vi "AnalyseFeRfe.vi"(6 "NISTData.NIDataArray":T2 {"Time Stamp" format="%^<%.3X\n%x>T"}, 8 "error in (no error)":errorcluster, 10 "Fluke":dbl[][](array[numeric]), 11 "NIST":dbl[][](array[numeric])) -> (0 "error out":errorcluster, 2 "Plot":cluster{dbl, "Time":dbl, dbl[][]}[](array[cluster]), 3 "FERfe Stats":dbl[][](array[numeric]))   [LabVIEW 2014]
uses:
  typedefs/NIDataArray.ctl
  typedefs/NIData.ctl
  typedefs/PhasorRectangular.ctl
  <vilib>/Analysis/6fits.llb/Curve Fitting Criteria.ctl
  <vilib>/measure/matone.llb/Extract Single Tone Information 1 Chan.vi
  <vilib>/Analysis/NI_AALPro.lvlib
  <vilib>/measure/NI_MAPro.lvlib
  <vilib>/Analysis/NI_AALBase.lvlib
panel:
  out "RFE Residual":T1(graph)
  out "FE Residual":T1(graph)
  out "RFE":cluster{dbl, "Time":dbl, dbl[][]}(graph)
  out "FE":cluster{dbl, "Time":dbl, dbl[][]}(graph)
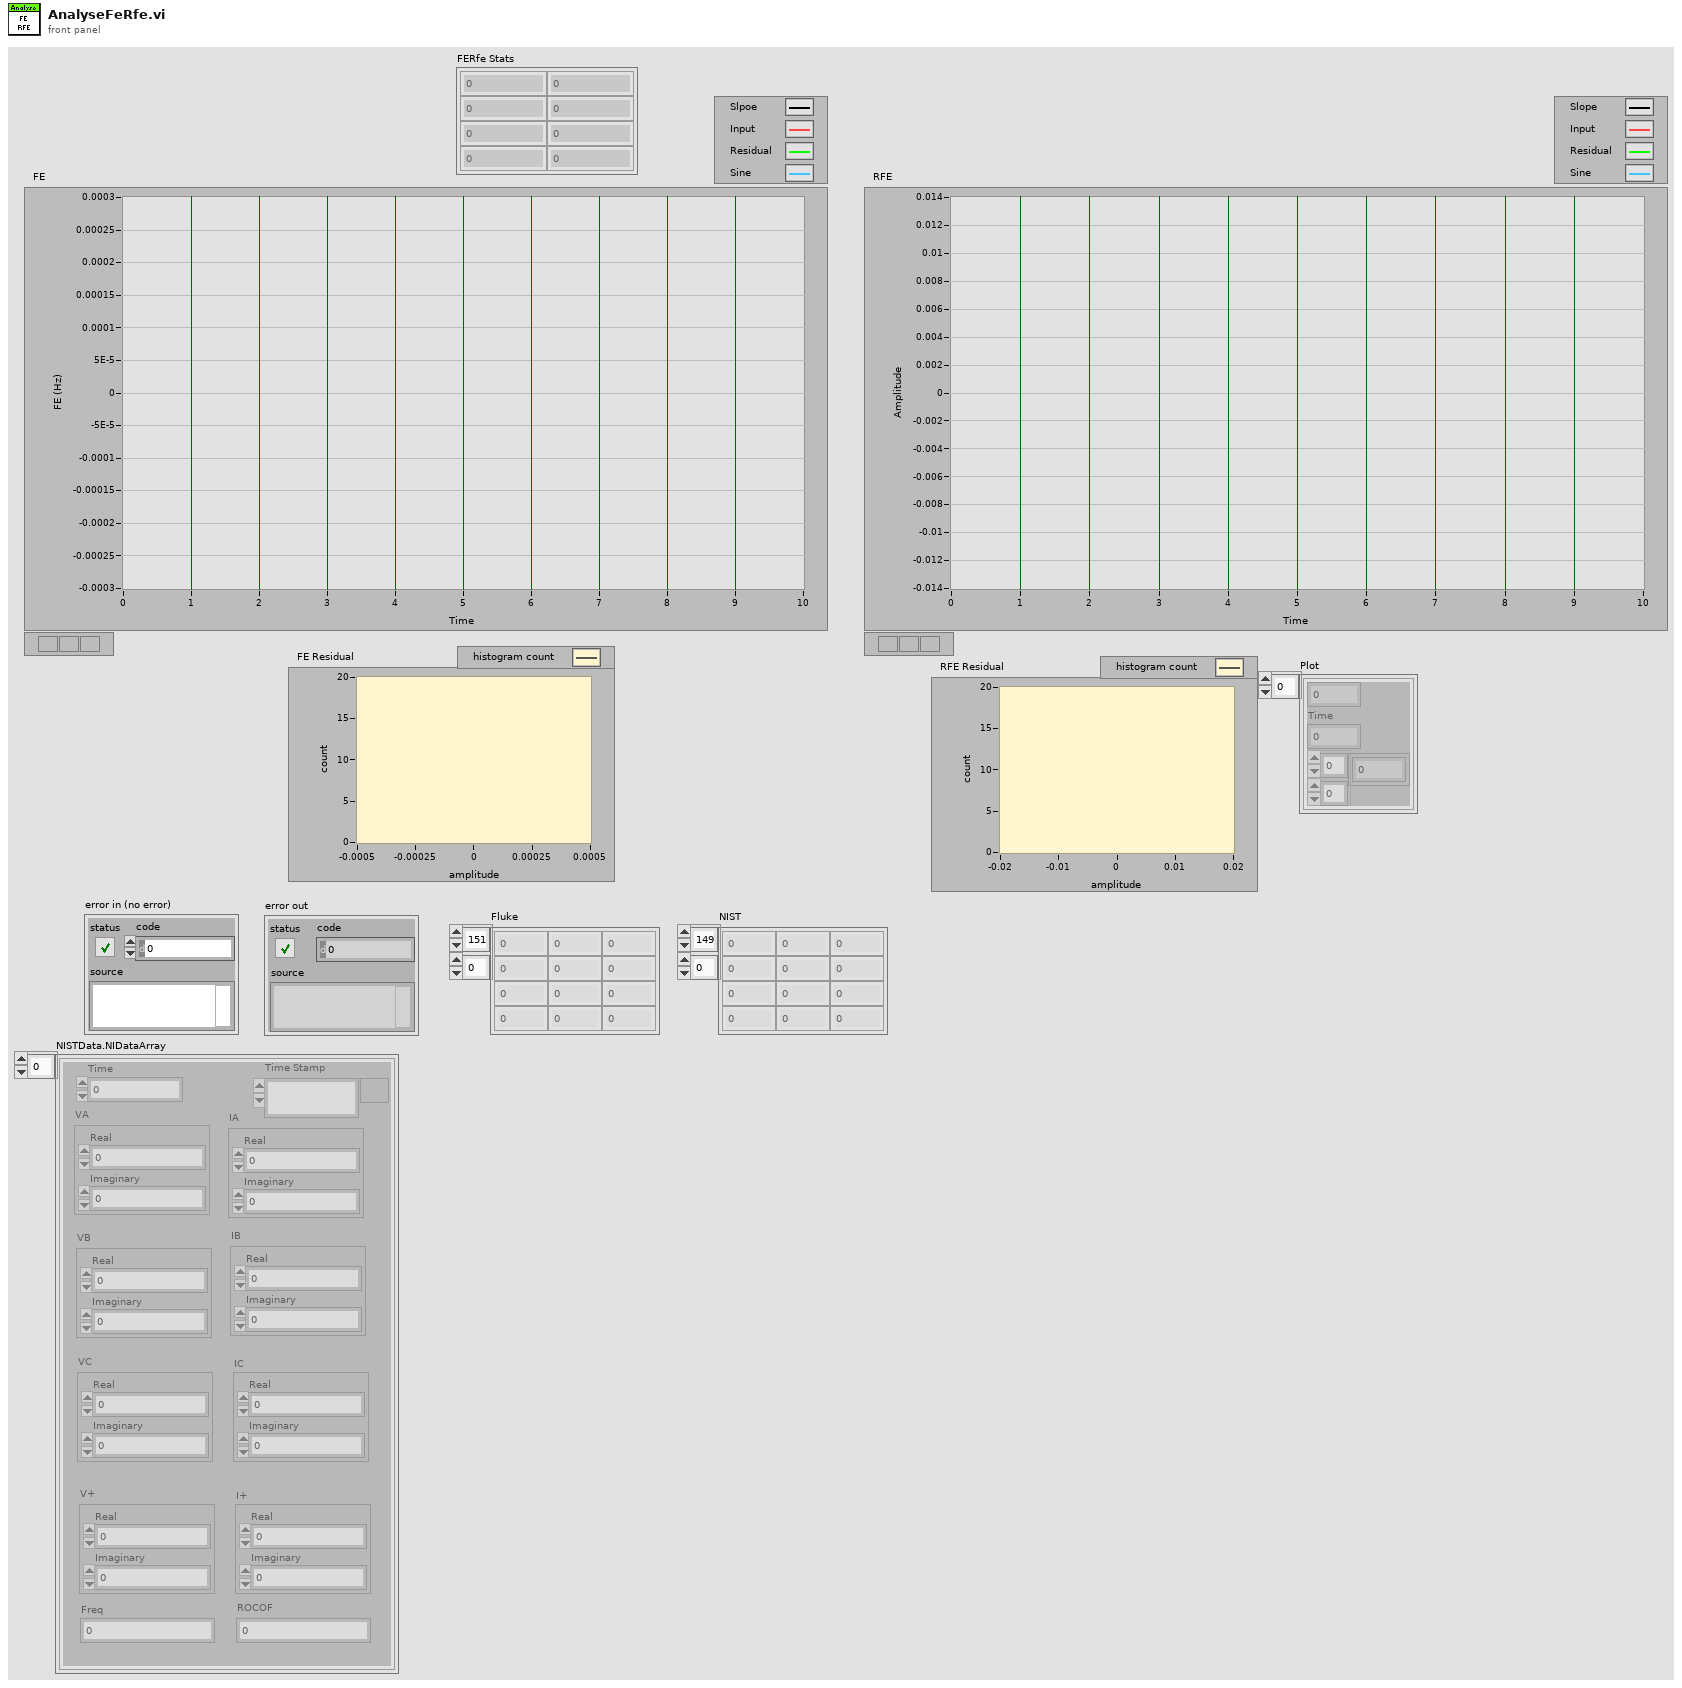
[diagram p1: front panel]
types:
  T1 = cluster{"X Values":dbl[], "Histogram: h(x)":i32[]}
  T2 = typedef "NIDataArray.ctl" = T3[]
  T3 = typedef "NIData.ctl" = cluster{"Time":dbl, "VA":T4, "VB":T4, "VC":T4, "V+":T4, "IA":T4, "IB":T4, "IC":T4, "I+":T4, "Freq":dbl, "ROCOF":dbl, "Time Stamp":timestamp}
  T4 = typedef "PhasorRectangular.ctl" = cluster{"Real":dbl, "Imaginary":dbl}
  T5 = enum32{"none", "input signal", "detected signal", "residual signal"}
  T6 = typedef "NI_AALPro.lvlib/Curve Fitting Criteria.ctl" = u16
  T7 = cluster{"exported time signal":waveform(dbl), "exported spectrum (dB)":cluster{"f0":dbl, "df":dbl, "dB Spectrum (Hann)":dbl[]}}
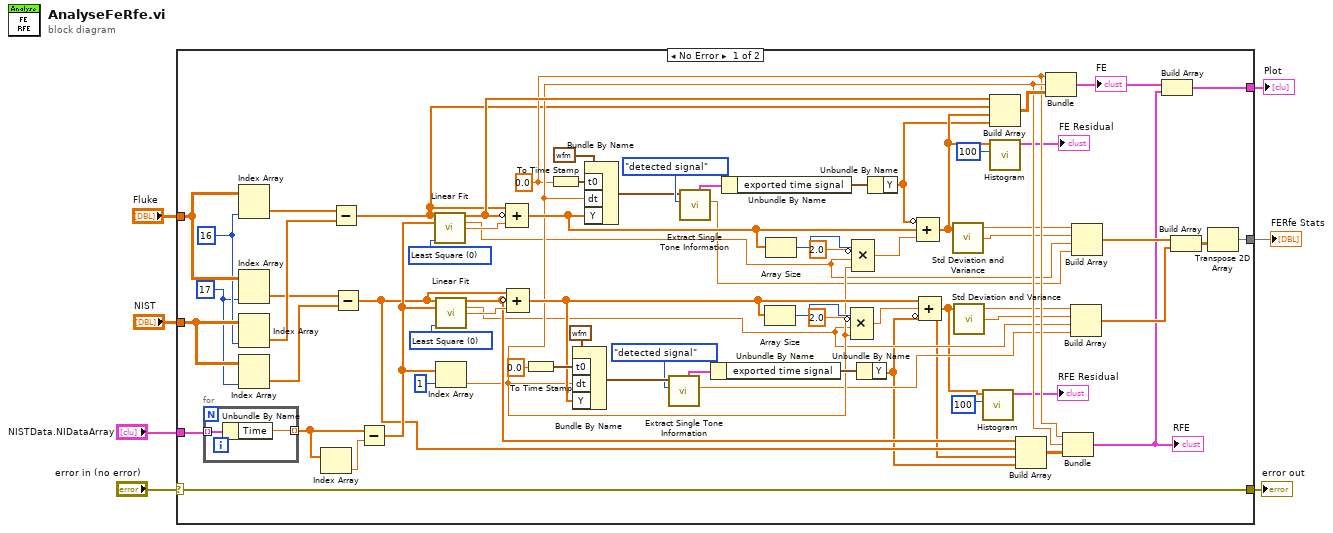
[diagram p0: block diagram]
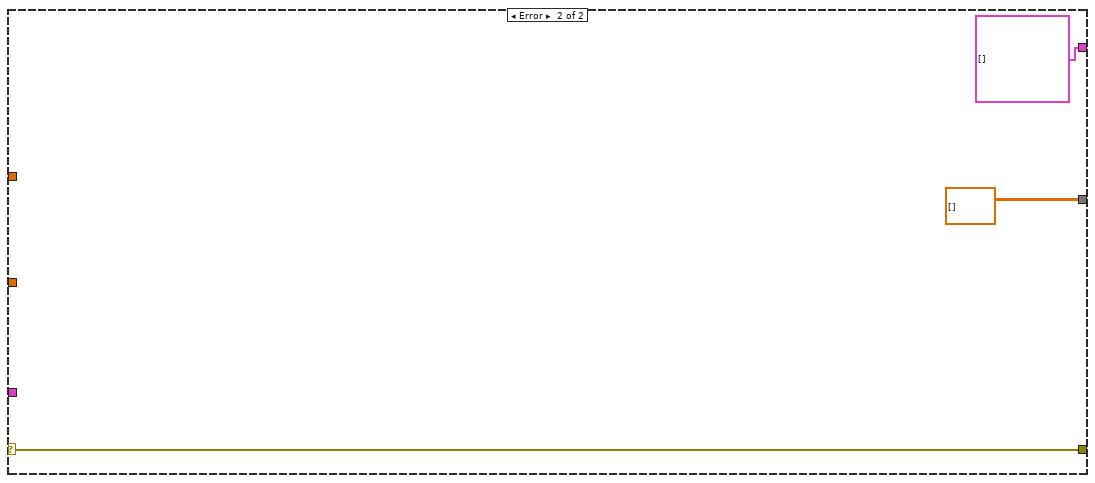
[diagram p2: hidden frame]
diagram:
  n1 = case shown="No Error" "error in (no error)" {
    selector: "error in (no error)" -> [w77 w82]
    tunnel: [w77 w82] -> w6
    tunnel: "NIST" -> [w75 _]
    tunnel: "Fluke" -> [w76 _]
    tunnel: "NISTData.NIDataArray" -> [w66 _]
    tunnel: [w14 dbl[][] []] -> w2
    tunnel: [w11 cluster{dbl, "Time":dbl, dbl[][]}[] []] -> w1
    frame No Error {
      w33 = 0.0
      w64 = T6 0 items=["Least Square", "Least Absolute Residual", "Bisquare"] ("method")
      w65 = T6 0 items=["Least Square", "Least Absolute Residual", "Bisquare"] ("method")
      w69 = 17 ("index")
      w70 = 16 ("index")
      n2 = for {
        tunnel: w66 -> [w79] mode=indexing
        tunnel: [w78] -> w67 mode=indexing
        n3 = Unbundle By Name(w79) -> ("Time"=w78:dbl)
      }
      n4 = Index Array(array=w76, index (col)=w70) -> (element=w74:dbl[])  [unwired: 1 in]
      n5 = Index Array(array=w76, index (col)=w69) -> (element=w72:dbl[])  [unwired: 1 in]
      n6 = Index Array(array=w75, index (col)=w70) -> (element=w73:dbl[])  [unwired: 1 in]
      n7 = Index Array(array=w75, index (col)=w69) -> (element=w71:dbl[])  [unwired: 1 in]
      n8 = Index Array(array=w67) -> (element=w68:dbl)  [unwired: 1 in]
      n9 = Subtract(x=w74, y=w73) -> (x-y=w18:dbl[])
      n10 = Subtract(x=w72, y=w71) -> (x-y=w17:dbl[])
      n11 = Subtract(x=w67, y=w68) -> (x-y=w61:dbl[])
      n12 = call <vilib>:"Linear Fit.vi"("Y"=w18, "X"=w61, "method"=w64) -> ("Best Linear Fit"=w38:dbl[], "slope"=w25:dbl, "intercept"=w63:dbl)  [unwired: 8 in, 2 out]
      n13 = call <vilib>:"Linear Fit.vi"("Y"=w17, "X"=w61, "method"=w65) -> ("Best Linear Fit"=w36:dbl[], "slope"=w21:dbl, "intercept"=w62:dbl)  [unwired: 8 in, 2 out]
      n14 = Index Array(array=w61, index=1) -> (element=w34:dbl)
      n15 = Compound Arithmetic op=ADD(w18, invert w38, w63) -> (w41:dbl[])
      n16 = Compound Arithmetic op=ADD(w17, invert w36, w62) -> (w42:dbl[])
      n17 = To Time Stamp(1:0.0) -> (0:w58:timestamp)
      n18 = To Time Stamp(1:w33) -> (0:w55:timestamp)
      n19 = Bundle By Name(cluster=waveform(dbl) {"t0"=timestamp(0 s since 1904-01-01), "dt"=1.0, "Y"=[]} ("time signal in"), "t0"=w58, "dt"=w34, "Y"=w42) -> (w54:waveform(dbl))
      n20 = Bundle By Name(cluster=waveform(dbl) {"t0"=timestamp(0 s since 1904-01-01), "dt"=1.0, "Y"=[]} ("time signal in"), "t0"=w55, "dt"=w34, "Y"=w41) -> (w47:waveform(dbl))
      n21 = call-poly <vilib>:"Extract Single Tone Information.vi"("export mode"=T5."detected signal", "time signal in"=w54) -> ("detected amplitude"=w20:dbl, "exported signals"=w52:T7)  [unwired: 4 in, 4 out]
      n22 = call-poly <vilib>:"Extract Single Tone Information.vi"("export mode"=T5."detected signal", "time signal in"=w47) -> ("detected amplitude"=w24:dbl, "exported signals"=w49:T7)  [unwired: 4 in, 4 out]
      n23 = Unbundle By Name(w52) -> ("exported time signal"=w51:waveform(dbl))
      n24 = Unbundle By Name(w49) -> ("exported time signal"=w50:waveform(dbl))
      n25 = Array Size(array=w42) -> (size(s)=w43:i32)
      n26 = Array Size(array=w41) -> (size(s)=w46:i32)
      n27 = Compound Arithmetic op=MULTIPLY(w43, invert 2.0 ("value"), w21, w34) -> (w39:dbl)
      n28 = Compound Arithmetic op=MULTIPLY(w46, invert 2.0 ("value"), w25, w34) -> (w40:dbl)
      n29 = Unbundle By Name(w51) -> ("Y"=w9:dbl[])
      n30 = Unbundle By Name(w50) -> ("Y"=w10:dbl[])
      n31 = Compound Arithmetic op=ADD(invert w10, w41, w40) -> (w32:dbl[])
      n32 = Compound Arithmetic op=ADD(w42, w39, invert w9) -> (w8:dbl[])
      n33 = call <vilib>:"Std Deviation and Variance.vi"("X"=w32) -> ("mean"=w27:dbl, "standard deviation"=w26:dbl)  [unwired: 1 in, 1 out]
      n34 = call <vilib>:"Std Deviation and Variance.vi"("X"=w8) -> ("mean"=w23:dbl, "standard deviation"=w22:dbl)  [unwired: 1 in, 1 out]
      n35 = call <vilib>:"Histogram.vi"("intervals"=100, "X"=w8) -> ("Histogram Graph"=→"RFE Residual":T1)  [unwired: 6 in, 3 out]
      n36 = Build Array(w38, w18, w32, w10) -> (w37:dbl[][])
      n37 = call <vilib>:"Histogram.vi"("intervals"=100, "X"=w32) -> ("Histogram Graph"=→"FE Residual":T1)  [unwired: 6 in, 3 out]
      n38 = Build Array(w36, w17, w8, w9) -> (w35:dbl[][])
      n39 = Bundle(w33, "Time"=w34, w37) -> (w13:cluster{dbl, "Time":dbl, dbl[][]})  [unwired: 1 in]
      "FE" <- w13
      n40 = Bundle(w33, "Time"=w34, w35) -> (w12:cluster{dbl, "Time":dbl, dbl[][]})  [unwired: 1 in]
      "RFE" <- w12
      n41 = Build Array(w23, w22, w21, w20) -> (w15:dbl[])
      n42 = Build Array(w27, w26, w25, w24) -> (w19:dbl[])
      n43 = Build Array(w13, w12) -> (w11:cluster{dbl, "Time":dbl, dbl[][]}[])
      n44 = Build Array(w19, w15) -> (w16:dbl[][])
      n45 = Transpose 2D Array(2D array=w16) -> (transposed array=w14:dbl[][])
    }
    frame Error {
    }
  }
  "error out" <- w6
  "FERfe Stats" <- w2
  "Plot" <- w1
